vi "queue-1.vi"() -> ()   [LabVIEW 2010]
panel:
  in  "send":bool
  in  "stop":bool
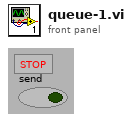
[diagram p1: front panel]
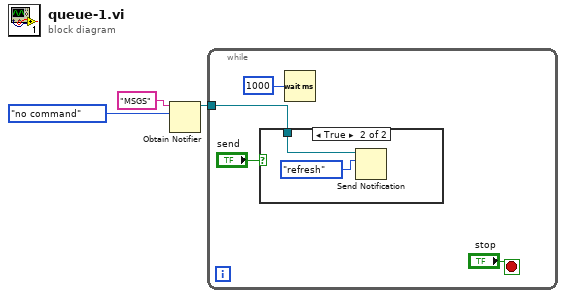
[diagram p0: block diagram]
diagram:
  n1 = Obtain Notifier(name (unnamed)="MSGS", notification data type=enum16{"no command", "refresh"}."no command") -> (notifier out=w1:refnum<notifier>)  [unwired: 2 in, 2 out]
  n2 = while {
    tunnel: w1 -> [w6]
    stop <- "stop" stop-if-true
    n3 = case shown="True" "send" {
      tunnel: w6 -> [_ w9]
      frame False {
      }
      frame True {
        n4 = Send Notification(notification=enum16{"no command", "refresh"}."refresh", notifier=w9) -> ()  [unwired: 1 in, 2 out]
      }
    }
    n5 = Wait (ms)(milliseconds to wait=u32 1000) -> ()  [unwired: 1 out]
  }
